vi "Append (Full) to filepath.vi"(11 "Filepath to Save Data":path) -> (3 "appended path":path)   [LabVIEW 2021]
doc: "Search and replace . with (Full). in the pathname"
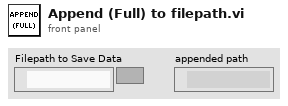
[diagram p1: front panel]
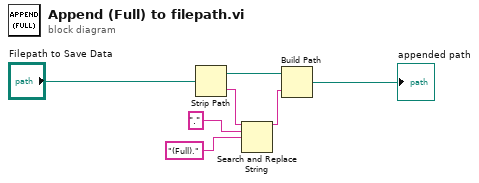
[diagram p0: block diagram]
diagram:
  n1 = Strip Path(path="Filepath to Save Data") -> (stripped path=w6:path, name=w2:string)
  n2 = Search and Replace String(input string=w2, search string=".", replace string="(Full)." ("replace string (\"\")")) -> (result string=w5:string)  [unwired: 5 in, 3 out]
  n3 = Build Path(base path=w6, name or relative path=w5) -> (appended path=→"appended path":path)
